vi "DrawValue.vi"(8 "start number?":bool, 9 "Value":i8, 10 "rect":T1, 11 "picture in":picture) -> (3 "picture out":picture)   [LabVIEW 2021, in "Cell.lvclass"]
uses:
  Cell.lvclass
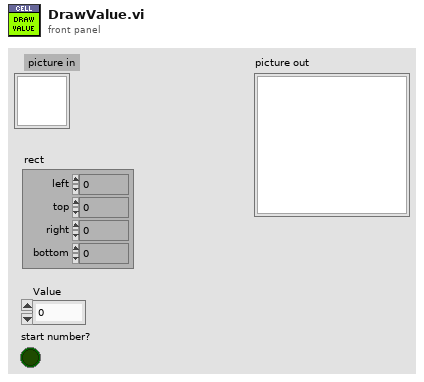
[diagram p1: front panel]
types:
  T1 = cluster{"left":i16, "top":i16, "right":i16, "bottom":i16}
  T2 = cluster{"Font Name:":string, "Size":i16, "Strikeout?":bool, "Italic?":bool, "Underline?":bool, "Outline?":bool, "Shadow?":bool, "Bold?":bool}
  T3 = enum16{"User-specified Font", "Application Font", "System Font", "Dialog Font"}
  T4 = cluster{"horizontal":enum16{"left", "center", "right"}, "vertical":enum16{"top", "center", "bottom"}}
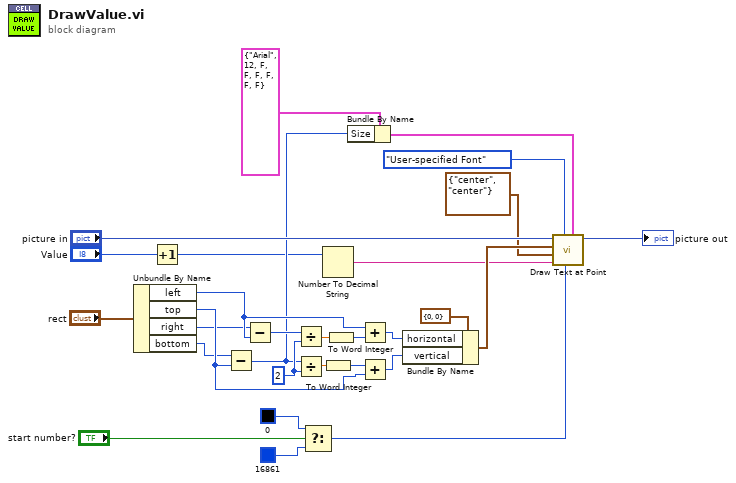
[diagram p0: block diagram]
diagram:
  w19 = i16 2 ("y")
  n1 = Unbundle By Name("rect") -> ("left"=w25:i16, "top"=w27:i16, "right"=w17:i16, "bottom"=w18:i16)
  n2 = Increment(x="Value") -> (x+1=w1:i8)
  n3 = Subtract(x=w18, y=w27) -> (x-y=w8:i16)
  n4 = Subtract(x=w17, y=w25) -> (x-y=w21:i16)
  n5 = Divide(x=w21, y=w19) -> (x/y=w23:dbl)
  n6 = Divide(x=w8, y=w19) -> (x/y=w22:dbl)
  n7 = Select(t=u32 0, s="start number?", f=u32 16861) -> (s? t:f=w2:u32)
  n8 = Number To Decimal String(number=w1) -> (decimal integer string=w6:string)  [unwired: 1 in]
  n9 = To Word Integer(number=w22) -> (16bit integer=w26:i16)
  n10 = To Word Integer(number=w23) -> (16bit integer=w24:i16)
  n11 = Bundle By Name(cluster=T2 {"Font Name:"="Arial", "Size"=12, "Strikeout?"=FALSE, "Italic?"=FALSE, "Underline?"=FALSE, "Outline?"=FALSE, "Shadow?"=FALSE, "Bold?"=FALSE} ("[user-specified font]"), "Size"=w8) -> (w9:T2)
  n12 = Add(x=w25, y=w24) -> (x+y=w28:i16)
  n13 = Add(x=w26, y=w27) -> (x+y=w29:i16)
  n14 = Bundle By Name(cluster=cluster{"horizontal":i16, "vertical":i16} {"horizontal"=0, "vertical"=0} ("origin(0,0)"), "horizontal"=w28, "vertical"=w29) -> (w13:cluster{"horizontal":i16, "vertical":i16})
  n15 = call <vilib>:"Draw Text at Point.vi"("[user-specified font]"=w9, "text color(black)"=w2, "desired font(Application)"=T3."User-specified Font", "text"=w6, "alignment(left, top)"=T4 {"horizontal"=enum."center", "vertical"=enum."center"}, "origin"=w13, "picture"="picture in") -> ("new picture"=→"picture out":picture)  [unwired: 3 in, 1 out]
